vi "数字量输出.vi"() -> ()   [LabVIEW 2015]
uses:
  <userlib>/DAQNavi Polymorphic VI/create/DAQNavi Create Channel(DO-Digital Output).vi
panel:
  out "error out 3":errorcluster
  in  "stop(true)":bool=TRUE
  out "error out 2":errorcluster caption="error out"
  in  "dataIn(U8Array)":u8[](array[numeric])
  out "error out":errorcluster
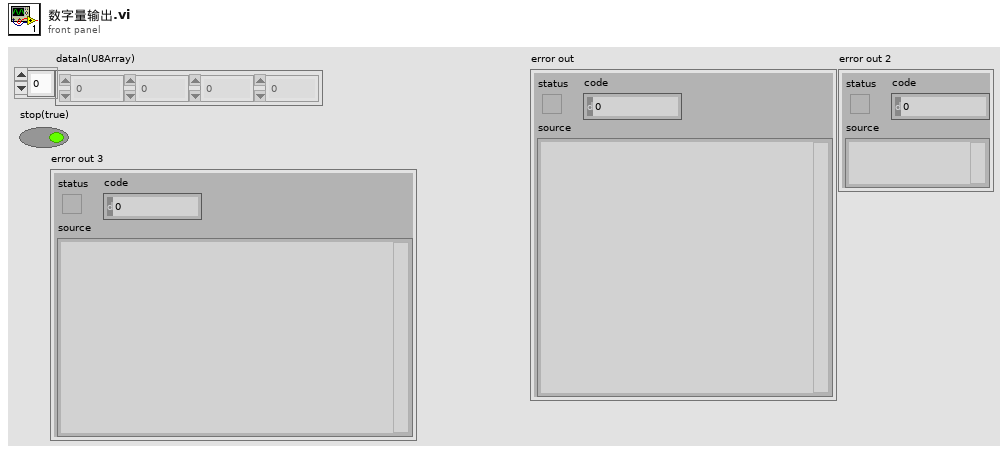
[diagram p1: front panel]
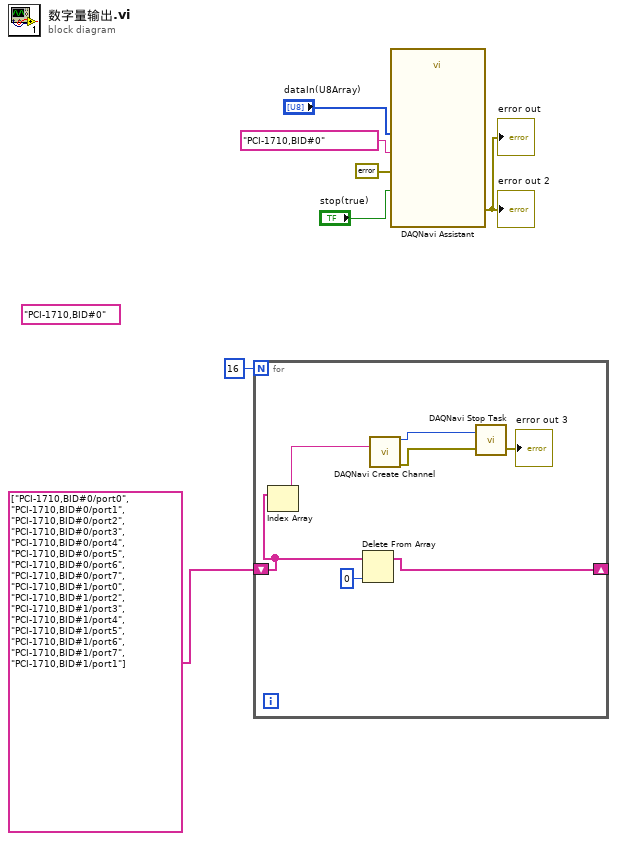
[diagram p0: block diagram]
diagram:
  (unwired) "PCI-1710,BID#0" ("physical channels")
  n1 = for {
    N: 16 -> [_]
    shift-right: [w8] -> _
    shift-left: string[] ["PCI-1710,BID#0/port0", "PCI-1710,BID#0/port1", "PCI-1710,BID#0/port2", "PCI-1710,BID#0/port3", "PCI-1710,BID#0/port4", "PCI-1710,BID#0/port5", "PCI-1710,BID#0/port6", "PCI-1710,BID#0/port7", "PCI-1710,BID#1/port0", "PCI-1710,BID#1/port2", "PCI-1710,BID#1/port3", "PCI-1710,BID#1/port4", "PCI-1710,BID#1/port5", "PCI-1710,BID#1/port6", "PCI-1710,BID#1/port7", "PCI-1710,BID#1/port1"] -> [w10]
    n2 = Index Array(array=w10) -> (element=w11:string)  [unwired: 1 in]
    n3 = Delete From Array(array=w10, index=0 ("索引")) -> (array with subset deleted=w8:string[])  [unwired: 1 in, 1 out]
    n4 = call-poly <userlib>:"DAQNavi Create Channel.vi"("physical channels"=w11) -> ("task out"=w14:i32, "error out"=w13:errorcluster)  [unwired: 13 in]
    n5 = call <userlib>:"DAQNavi Stop Task.vi"("error in (no error)"=w13, "task in"=w14) -> ("error out"=→"error out 3":errorcluster)  [unwired: 1 out]
  }
  n6 = call "DAQNavi Assistant"("error in(no error)"=errorcluster {"status"=FALSE, "code"=0, "source"=""}, "stop(true)"="stop(true)", "dataIn(U8Array)"="dataIn(U8Array)", "device description"="PCI-1710,BID#0" ("physical channels")) -> ("error out"=→"error out" →"error out 2":errorcluster)  [unwired: 23 in]
